vi "Calculate Rectangle.vi"(8 "error in (no error)":errorcluster, 11 "FSM.Node in":refnum<class "FSM.Node.lvclass">) -> (0 "error out":errorcluster, 3 "FSM.Node out":refnum<class "FSM.Node.lvclass">)   [LabVIEW 2015, in "FSM.Node.lvclass"]
uses:
  FSM.Node.lvclass
  FSM.Node.lvclass/FSM.Node.ctl
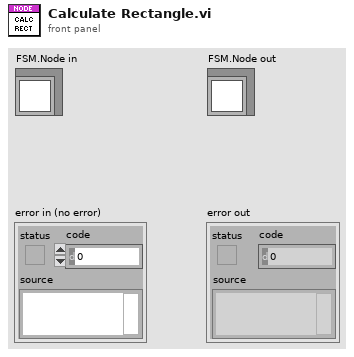
[diagram p1: front panel]
types:
  T1 = typedef "FSM.Node.lvclass/Shape.ctl" = enum16{"Default", "Start", "Action", "End"}
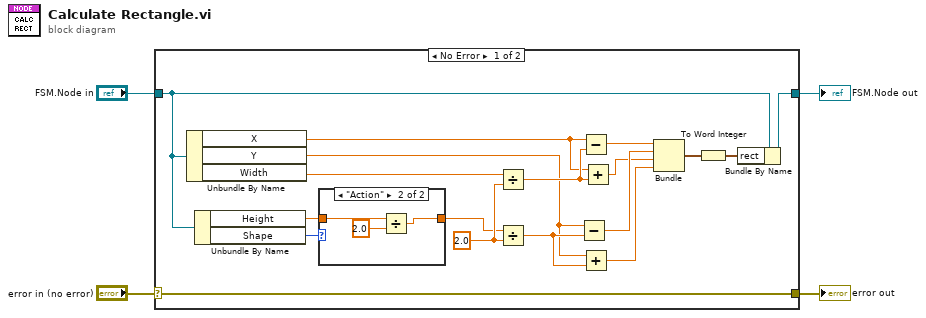
[diagram p0: block diagram]
diagram:
  n1 = case shown="No Error" "error in (no error)" {
    selector: "error in (no error)" -> [w22 w28]
    tunnel: [w22 w28] -> w3
    tunnel: [w9 w27] -> w1
    tunnel: "FSM.Node in" -> [w8 w27]
    frame No Error {
      w20 = 2.0
      n2 = Unbundle By Name(w8) -> ("X"=w12:dbl, "Y"=w11:dbl, "Width"=w21:dbl)
      n3 = Unbundle By Name(w8) -> ("Height"=w6:dbl, "Shape"=w7:T1)
      n4 = case shown="\"Action\"" w7 {
        tunnel: w6 -> [w23 w26]
        tunnel: [w23 w25] -> w5
        frame "Default", Default {
        }
        frame "Action" {
          n5 = Divide(x=w26, y=2.0) -> (x/y=w25:dbl)
        }
      }
      n6 = Divide(x=w21, y=w20) -> (x/y=w19:dbl)
      n7 = Divide(x=w5, y=w20) -> (x/y=w18:dbl)
      n8 = Subtract(x=w11, y=w18) -> (x-y=w14:dbl)
      n9 = Subtract(x=w12, y=w19) -> (x-y=w15:dbl)
      n10 = Add(x=w11, y=w18) -> (x+y=w17:dbl)
      n11 = Add(x=w12, y=w19) -> (x+y=w13:dbl)
      n12 = Bundle(w15, w14, w13, w17) -> (w16:cluster{dbl, dbl, dbl, dbl})  [unwired: 1 in]
      n13 = To Word Integer(number=w16) -> (16bit integer=w10:cluster{i16, i16, i16, i16})
      n14 = Bundle By Name(cluster=w8, "rect"=w10) -> (w9:refnum<class "FSM.Node.lvclass">)
    }
    frame Error {
    }
  }
  "error out" <- w3
  "FSM.Node out" <- w1
